vi "GetSingleAiChan.vi"(8 "TimeOut (ms)":i32=1000, 9 "ChanSel":i16, 10 "Num":u32=1000 caption="PtsToRead", 11 "error in":errorcluster caption="错误输入") -> (0 "Data":sgl[](array[numeric]), 3 "error out":errorcluster caption="错误输出")   [LabVIEW 2016]
uses:
  PLC-Lab/lib/gusb.dll
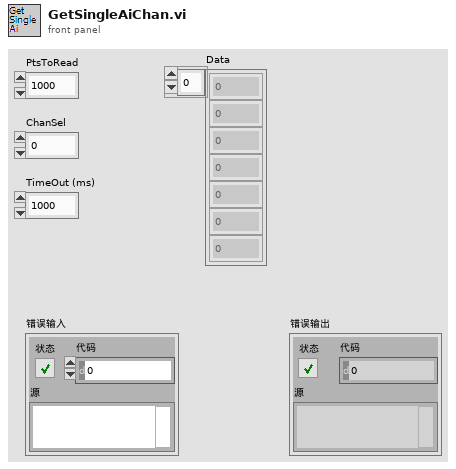
[diagram p1: front panel]
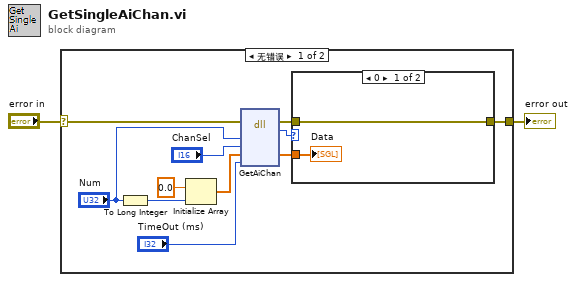
[diagram p0: block diagram]
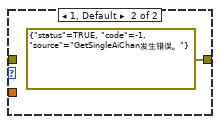
[diagram p2: hidden frame]
diagram:
  n1 = case shown="无错误" "error in" {
    selector: "error in" -> [w13 w17]
    tunnel: [w7 w17] -> w1
    frame No Error {
      n2 = To Long Integer(number="Num") -> (32bit integer=w4:i32)
      n3 = Initialize Array(sgl 0.0 ("元素"), w4) -> (w10:sgl[])
      n4 = dll-call lib="E:/Camproject/2018/2018.1Labview/PLC-Lab/lib/gusb.dll" fn="GetAiChan"(error in=w13, "Num"="Num", "ChanSel"="ChanSel", "Buf"=w10, "TimeOut"="TimeOut (ms)") -> (error out=w8:errorcluster, "Status"=w6:i32, "Buf"=w3:sgl[])  [unwired: 5 in, 1 out]
      n5 = case shown="0" w6 {
        tunnel: w8 -> [w15 _]
        tunnel: [w15 errorcluster {"status"=TRUE, "code"=-1, "source"="GetSingleAiChan发生错误。"} ("错误常量")] -> w7
        tunnel: w3 -> [w14 _]
        frame 0 {
          "Data" <- w14
        }
        frame 1, Default {
        }
      }
    }
    frame Error {
    }
  }
  "error out" <- w1
